vi "Send Message.vi"(8 "error in (no error)":errorcluster, 9 "Data":string, 10 "ID":string, 11 "Websocket Client in":refnum<class "Websocket Client.lvclass">) -> (0 "error out":errorcluster, 3 "Websocket Client out":refnum<class "Websocket Client.lvclass">)   [LabVIEW 2020]
uses:
  Websocket Client.lvclass/Websocket Client.ctl
  Websocket Client.lvclass
  C:/Program Files (x86)/National Instruments/LabVIEW 2020/vi.lib/IlluminatedG/lv-stream/Connection/Connection.lvclass
  C:/Program Files (x86)/National Instruments/LabVIEW 2020/vi.lib/IlluminatedG/lv-stream/Endpoint/Endpoint.lvclass
  C:/dev/IlluminatedG/lv-stream-websocket/Stream-Websocket/Websocket Client/Websocket Client.lvclass
  WebsocketStream/WebsocketStream.lvclass
  C:/Program Files (x86)/National Instruments/LabVIEW 2020/vi.lib/IlluminatedG/lv-stream/stream/Stream.lvclass
  C:/dev/IlluminatedG/lv-stream-websocket/Stream-Websocket/WebsocketStream/WebsocketStream.lvclass
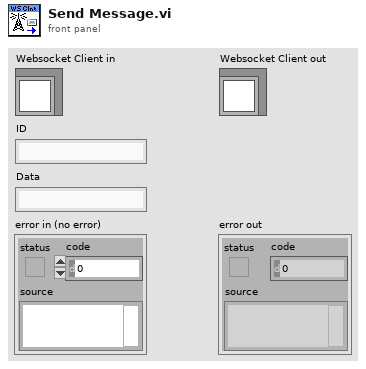
[diagram p1: front panel]
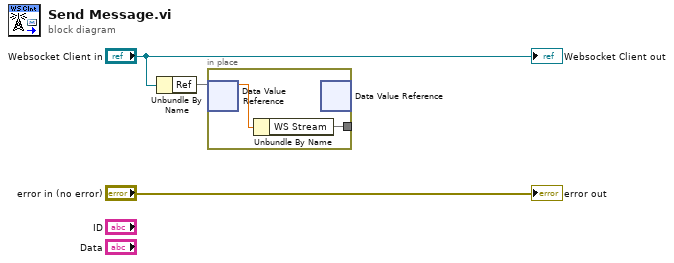
[diagram p0: block diagram]
diagram:
  n1 = Unbundle By Name("Websocket Client in") -> ("Ref"=w2)
  n2 = in-place {
    in-place-border: [w4] -> _
    n3 = in-place-dvr #1(w2) -> (w5:dbl)  [unwired: 1 out]
    n4 = Unbundle By Name(w5) -> ("WS Stream"=w4)
    n5 = in-place-dvr #1() -> ()  [unwired: 1 in, 2 out]
  }
  "error out" <- "error in (no error)"
  "Websocket Client out" <- "Websocket Client in"
